vi "Media si dispersia Metoda 1.vi"() -> ()   [LabVIEW 2011]
panel:
  in  "Boolean":bool
  out "Suma celor N nr. aleatorii":dbl
  out "Dispersia":dbl
  out "Media":dbl
  out "Sir ce are ultima valoare Suma":dbl[](array[numeric]) format="%#.3g"
  out "Sir cu N nr. aleatorii":dbl[](array[numeric]) format="%#.3g"
  in  "N nr. aleatorii":u8
  # "Suma"
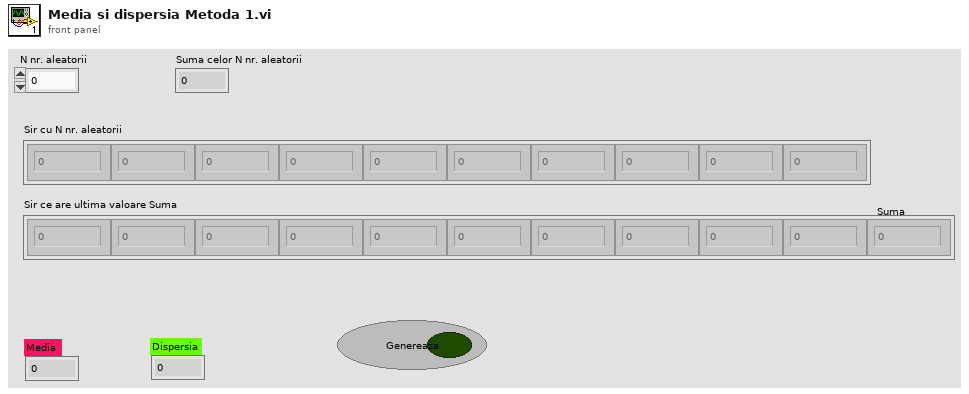
[diagram p1: front panel]
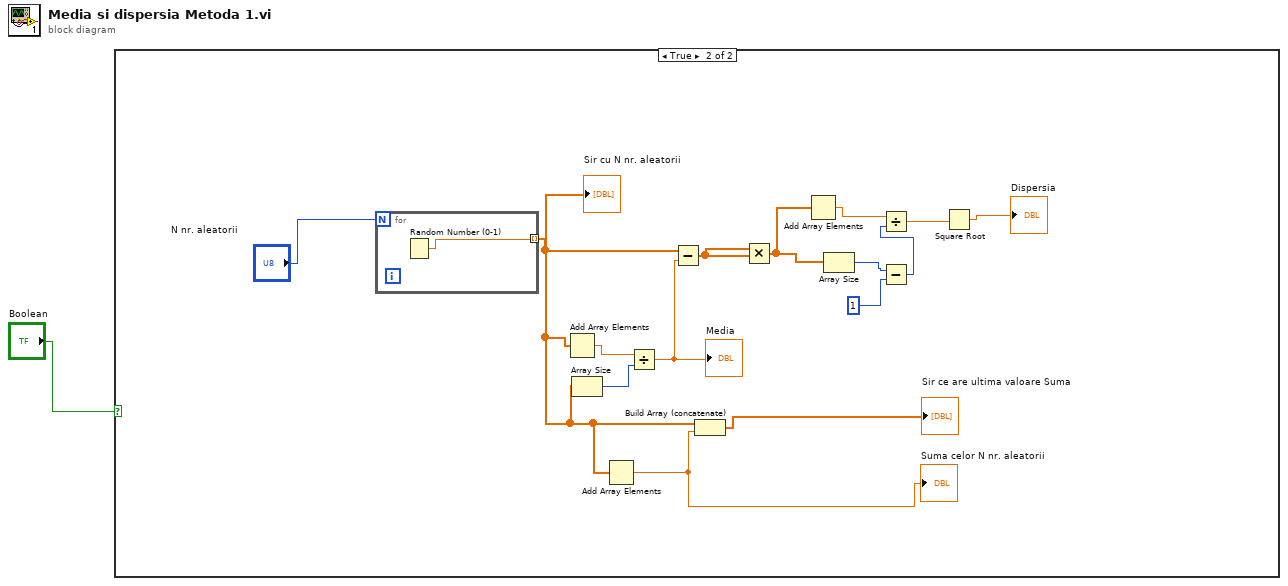
[diagram p0: block diagram]
diagram:
  n1 = case shown="True" "Boolean" {
    frame False {
    }
    frame True {
      n2 = for {
        N: "N nr. aleatorii" -> [_]
        tunnel: [w17] -> w8 mode=indexing
        n3 = Random Number (0-1)() -> (number: 0 to 1=w17:dbl)
      }
      "Sir cu N nr. aleatorii" <- w8
      n4 = Add Array Elements(numeric array=w8) -> (sum=w6:dbl)
      n5 = Array Size(array=w8) -> (size(s)=w7:i32)
      n6 = Add Array Elements(numeric array=w8) -> (sum=w5:dbl)
      "Suma celor N nr. aleatorii" <- w5
      n7 = Divide(x=w6, y=w7) -> (x/y=w9:dbl)
      "Media" <- w9
      n8 = Subtract(x=w8, y=w9) -> (x-y=w10:dbl[])
      n9 = Build Array (concatenate) "Build Array"(w8, w5) -> (→"Sir ce are ultima valoare Suma":dbl[])
      n10 = Multiply(x=w10, y=w10) -> (x*y=w2:dbl[])
      n11 = Add Array Elements(numeric array=w2) -> (sum=w11:dbl)
      n12 = Array Size(array=w2) -> (size(s)=w14:i32)
      n13 = Subtract(x=w14, y=1) -> (x-y=w16:i32)
      n14 = Divide(x=w11, y=w16) -> (x/y=w12:dbl)
      n15 = Square Root(x=w12) -> (sqrt(x)=→"Dispersia":dbl)
    }
  }
